vi "Launch MiniGUIs.vi"(8 "error in (no error)":errorcluster, 11 "LabGUI in":refnum<class "LabGUI.lvclass">) -> (0 "error out":errorcluster, 3 "LabGUI out":refnum<class "LabGUI.lvclass">)   [LabVIEW 2019]
uses:
  <vilib>/MGI/Panel Manager/Panel Actor/Panel Actor/Panel Actor.lvclass
  <vilib>/MGI/Panel Manager/Panel/Panel.lvlib
  <vilib>/MGI/Panel Manager/Panel/Panel/Subpanel/Subpanel.vi
  <vilib>/MGI/Panel Manager/Panel/Panel/Subpanel/Subpanel.lvclass
  MiniGUI/MiniGUI/MiniGUI.lvclass
  LabGUI.lvclass
  C:/Program Files (x86)/National Instruments/LabVIEW 2019/vi.lib/MGI/Panel Manager/Panel Actor/Panel Actor/Panel Actor.lvclass
  C:/Program Files (x86)/National Instruments/LabVIEW 2019/vi.lib/MGI/Monitored Actor/Monitored Actor/Monitored Actor/Monitored Actor.lvclass
  C:/Program Files (x86)/National Instruments/LabVIEW 2019/vi.lib/ActorFramework/Actor/Actor.lvclass
  C:/Program Files (x86)/National Instruments/LabVIEW 2019/vi.lib/MGI/Panel Manager/Panel/Panel/Panel.lvclass
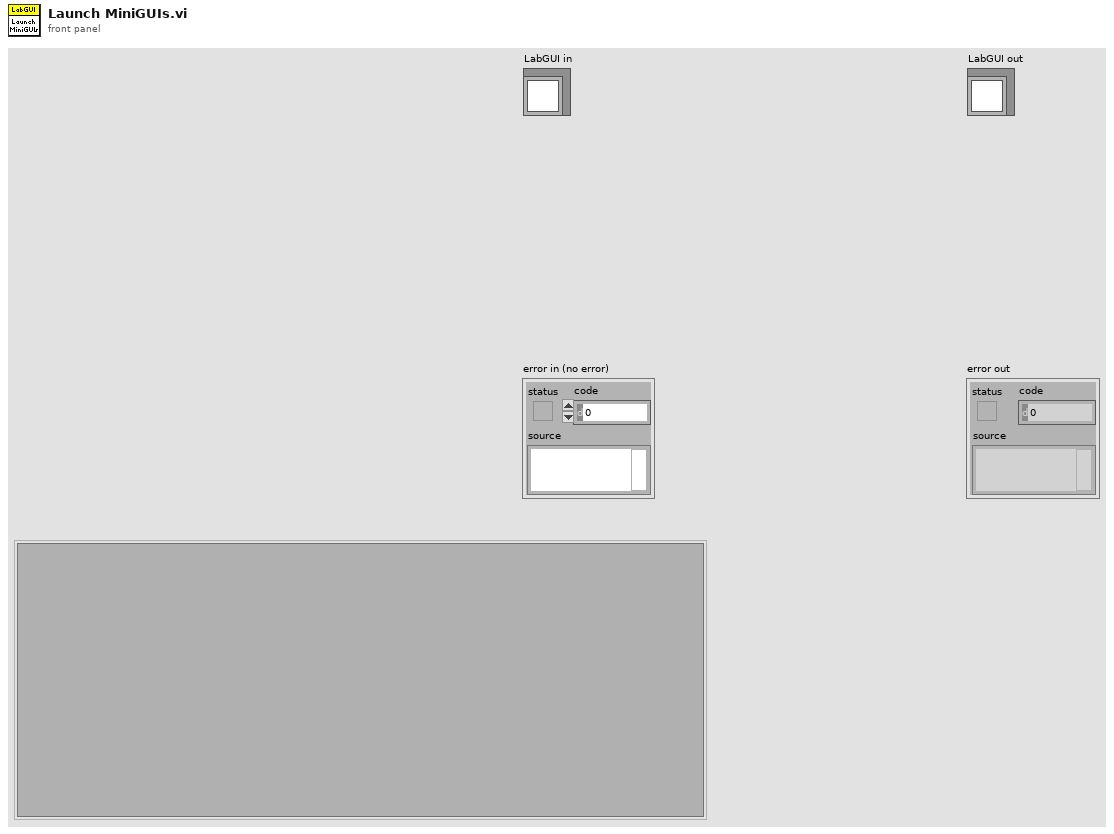
[diagram p1: front panel]
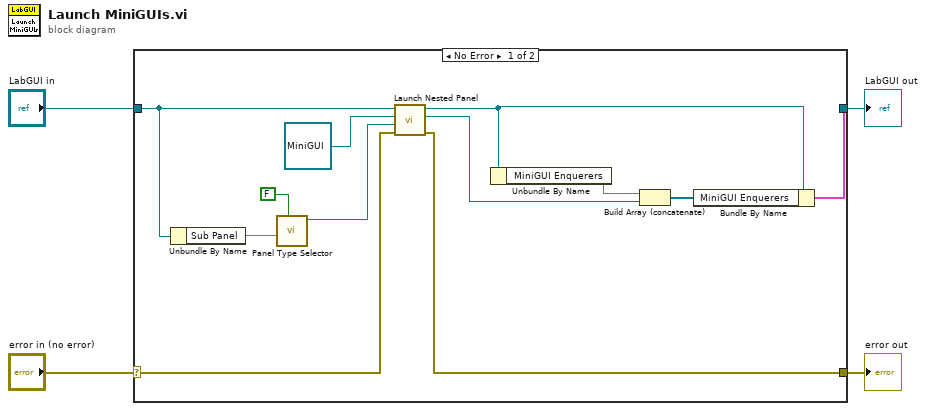
[diagram p0: block diagram]
diagram:
  n1 = case shown="No Error" "error in (no error)" {
    selector: "error in (no error)" -> [w16 w18]
    tunnel: [w15 w18] -> w3
    tunnel: [w6 w17] -> w1
    tunnel: "LabGUI in" -> [w9 w17]
    frame No Error {
      n2 = Unbundle By Name(w9) -> ("Sub Panel"=w12)
      n3 = call-poly <vilib>:"Panel Type Selector.vi"("Autoshow? (T)"=FALSE, "Sub Panel"=w12) -> ("Subpanel Out"=w13:refnum<class "Subpanel.lvclass">)  [unwired: 8 in, 1 out]
      n4 = call <vilib>:"Launch Nested Panel.vi"("error in (no error)"=w16, "Panel"=w13, "Nested Panel Actor"=refnum<class "MiniGUI.lvclass"> refnum ("MiniGUI Actor.lvlib:MiniGUI.lvclass"), "Panel Actor in"=w9) -> ("error out"=w15:errorcluster, "Nested Actor's Enqueuer"=w8:refnum<class "Message Enqueuer.lvclass">, "Panel Actor out"=w7:refnum<class "LabGUI.lvclass">)  [unwired: 4 in, 1 out]
      n5 = Unbundle By Name(w7) -> ("MiniGUI Enquerers"=w10)
      n6 = Build Array (concatenate)(w10, w8) -> (w5:refnum<class "Message Enqueuer.lvclass">[])
      n7 = Bundle By Name(cluster=w7, "MiniGUI Enquerers"=w5) -> (w6:cluster{})
    }
    frame Error {
    }
  }
  "error out" <- w3
  "LabGUI out" <- w1
